vi "Rotation2d_RotateBy.vi"(9 "other Rotation":T1 {"SIN" format="%13.4f"; "COS" format="%13.4f"; "VALUE" format="%13.4f"}, 11 "in ROTATION":T1 {"SIN" format="%13.4f"; "COS" format="%13.4f"; "VALUE" format="%13.4f"}) -> (3 "out ROTATION":T1 {"SIN" format="%13.4f"; "COS" format="%13.4f"; "VALUE" format="%13.4f"})   [LabVIEW 2019, in "Trajectory_Library.lvlib"]
doc: "Adds the new rotation to the current rotation using a rotation matrix.\n\nThe matrix multiplication is as follows:\n [cos_new] [other.cos, -other.sin][cos]\n [sin_new] = [other.sin, other.cos][sin]\n value_new = atan2(cos_new, sin_new)\n\nThis is the same as Plus.\n\nParameters:\n - IN ROTATION - This ROTATION data structure\n - OTHER ROTATION - The rotation to rotate by\n\nReturns:\n - OUT ROTATION - The new rotated Rotation2d."
uses:
  Trajectory_Library.lvlib
  ROTATION2D.ctl
  Util_CalcDist.vi
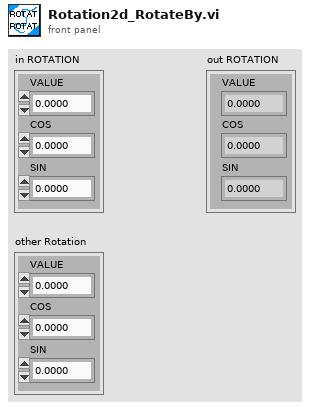
[diagram p1: front panel]
types:
  T1 = typedef "Trajectory_Library.lvlib/ROTATION2D.ctl" = cluster{"VALUE":dbl, "COS":dbl, "SIN":dbl}
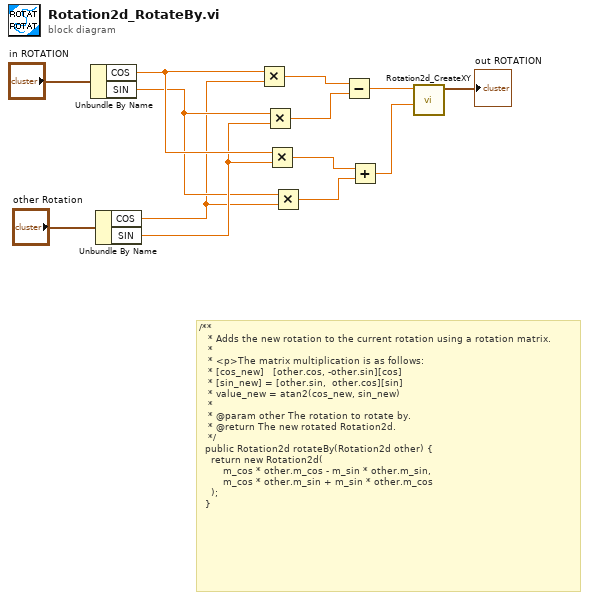
[diagram p0: block diagram]
diagram:
  # "/**\n   * Adds the new rotation to the current rotation using a rotation matrix.\n   *\n   * <p>The matrix multiplication is as follows:\n   * [cos_new]   [other.cos, -other.sin][cos]\n   * [sin_new] = [other.sin,  other.cos][sin]\n   * value_new = atan2(cos_new, sin_new)\n   *\n   * @param other The rotation to rotate by.\n   * @return The new rotated Rotation2d.\n   */\n  public Rotation2d rotateBy(Rotation2d other) {\n    return new Rotation2d(\n        m_cos * other.m_cos - m_sin * other.m_sin,\n        m_cos * other.m_sin + m_sin * other.m_cos\n    );\n  }"
  n1 = Unbundle By Name("in ROTATION") -> ("COS"=w8:dbl, "SIN"=w6:dbl)
  n2 = Unbundle By Name("other Rotation") -> ("COS"=w5:dbl, "SIN"=w7:dbl)
  n3 = Multiply(x=w8, y=w5) -> (x*y=w12:dbl)
  n4 = Multiply(x=w6, y=w7) -> (x*y=w11:dbl)
  n5 = Multiply(x=w8, y=w7) -> (x*y=w10:dbl)
  n6 = Multiply(x=w6, y=w5) -> (x*y=w9:dbl)
  n7 = Subtract(x=w12, y=w11) -> (x-y=w2:dbl)
  n8 = Add(x=w10, y=w9) -> (x+y=w1:dbl)
  n9 = call "Rotation2d_CreateXY.vi"("Y or sine"=w1, "X or  cosine"=w2) -> ("ROTATION"=→"out ROTATION":T1)  [unwired: 9 in]
